vi "SetGobjectPose.vi"(2 "contents":string, 3 "Object in":refnum<vi>) -> (0 "remaining":string, 1 "Object out":refnum<vi>)   [LabVIEW 2010]
uses:
  <vilib>/picture/3D Picture Control/NI_3D Picture Control.lvlib
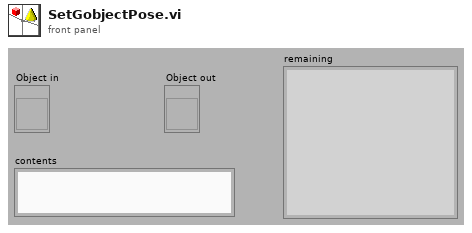
[diagram p1: front panel]
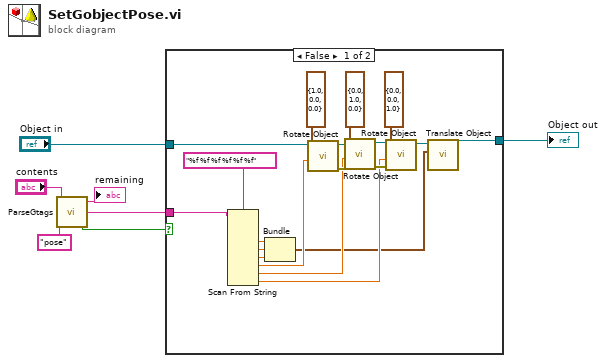
[diagram p0: block diagram]
diagram:
  n1 = call "ParseGtags.vi"("tag"="pose", "urdf in"="contents") -> ("not found"=w1:bool, "contents"=w2:string, "urdf out"=→"remaining":string)  [unwired: 1 out]
  n2 = case shown="False" w1 {
    tunnel: [w10 w27] -> w7
    tunnel: "Object in" -> [w9 w27]
    tunnel: w2 -> [w12 _]
    frame False {
      n3 = Scan From String(format string="%f %f %f %f %f %f", input string=w12) -> (output 1=w21:dbl, output 2=w19:dbl, output 3=w20:dbl, output 4=w18:dbl, output 5=w17:dbl, output 6=w16:dbl)  [unwired: 8 in, 3 out]
      n4 = Bundle(w21, w19, w20) -> (w8:cluster{dbl, dbl, dbl})  [unwired: 1 in]
      n5 = call <vilib>:"Rotate Object.vi"("Angle"=w18, "Axis"=cluster{"X":sgl, "Y":sgl, "Z":sgl} {"X"=1.0, "Y"=0.0, "Z"=0.0}, "Scene.Object In"=w9) -> ("error out"=w23:errorcluster, "Scene.Object Out"=w24:refnum<vi>)  [unwired: 7 in]
      n6 = call <vilib>:"Rotate Object.vi"("error in (no error)"=w23, "Angle"=w17, "Axis"=cluster{"X":sgl, "Y":sgl, "Z":sgl} {"X"=0.0, "Y"=1.0, "Z"=0.0}, "Scene.Object In"=w24) -> ("error out"=w25:errorcluster, "Scene.Object Out"=w26:refnum<vi>)  [unwired: 6 in]
      n7 = call <vilib>:"Rotate Object.vi"("error in (no error)"=w25, "Angle"=w16, "Axis"=cluster{"X":sgl, "Y":sgl, "Z":sgl} {"X"=0.0, "Y"=0.0, "Z"=1.0}, "Scene.Object In"=w26) -> ("Scene.Object Out"=w11:refnum<vi>)  [unwired: 6 in, 1 out]
      n8 = call <vilib>:"Translate Object.vi"("Translation"=w8, "Scene.Object In"=w11) -> ("Scene.Object Out"=w10:refnum<vi>)  [unwired: 8 in, 1 out]
    }
    frame True {
    }
  }
  "Object out" <- w7
